vi "String Width.vi"(11 "string":string) -> (3 "string width":i32)   [LabVIEW 2017]
doc: "Calculates the <b>string</b> width after conversion into picture."
uses:
  Settings/Default Settings.vi
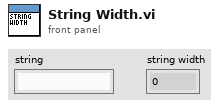
[diagram p1: front panel]
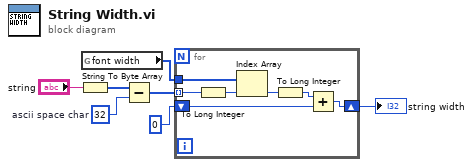
[diagram p0: block diagram]
diagram:
  w5 = u8 32  # ascii space char
  n1 = String To Byte Array(string="string") -> (unsigned byte array=w6:u8[])
  n2 = global read "Default Settings.vi" "font width"() -> (w3:i16[])
  n3 = Subtract(x=w6, y=w5) -> (x-y=w4:u8[])
  n4 = for {
    tunnel: w4 -> [w13] mode=indexing
    tunnel: w3 -> [w14]
    shift-right: [w10] -> w1
    shift-left: 0 -> [w9]
    n5 = To Long Integer(number=w13) -> (32bit integer=w12:i32)
    n6 = Index Array(array=w14, index=w12) -> (element=w11:i16)
    n7 = To Long Integer(number=w11) -> (32bit integer=w8:i32)
    n8 = Add(x=w8, y=w9) -> (x+y=w10:i32)
  }
  "string width" <- w1
